vi "main-aq-program.vi"() -> ()   [LabVIEW 2015]
uses:
  <vilib>/userdefined/High Color/IMAQdx.ctl
  globals.vi
  <vilib>/vision/driver/NI_Vision_Acquisition_Software.lvlib
  <resource>/objmgr/imaqdx.rc
panel:
  in  "Save image":bool
  in  "Name":string
  in  "Path":path
  out "Image 2":T1(plugin-control)
  out "Image":T1(plugin-control)
  in  "Camera-right":T2="cam4"
  in  "Exposure time left":dbl=10000.0
  in  "Stop Button":bool
  in  "Camera-left":T2="cam4"
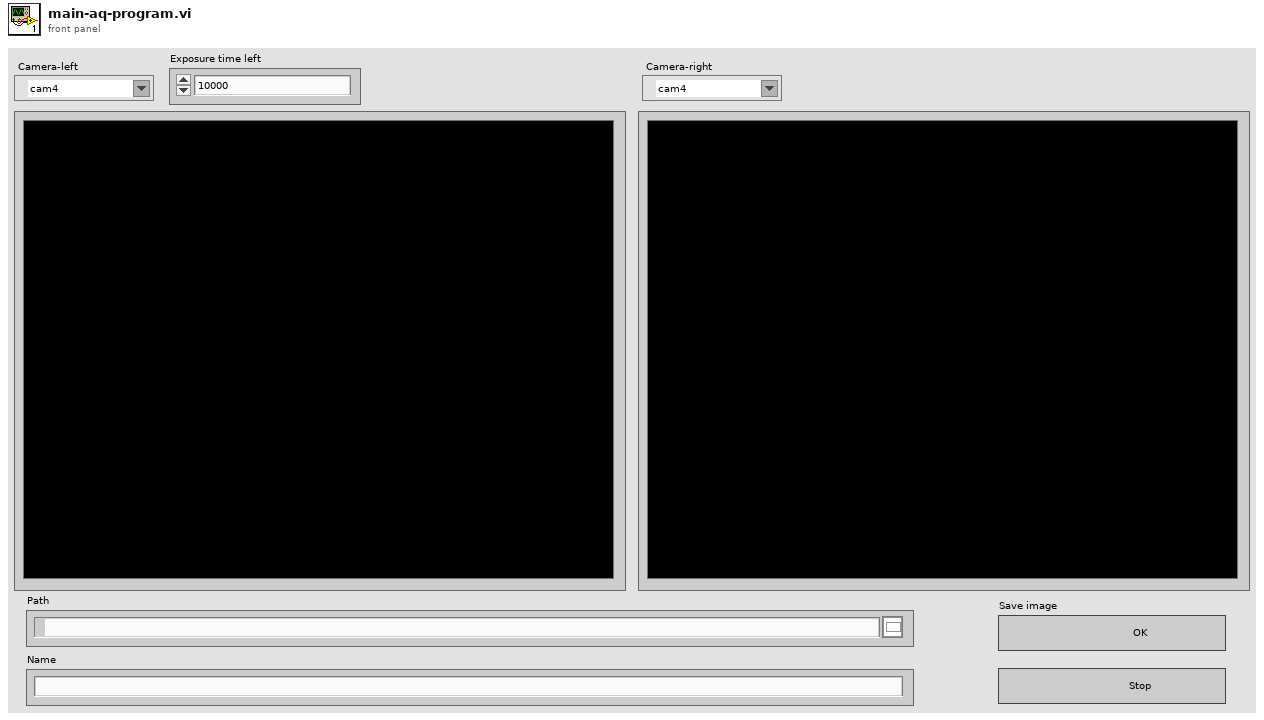
[diagram p1: front panel]
types:
  T1 = typedef "IMAQ Image.ctl" = refnum<image>
  T2 = typedef "IMAQdx.ctl" = refnum<k21>
  T3 = typedef "Image Type" = u32
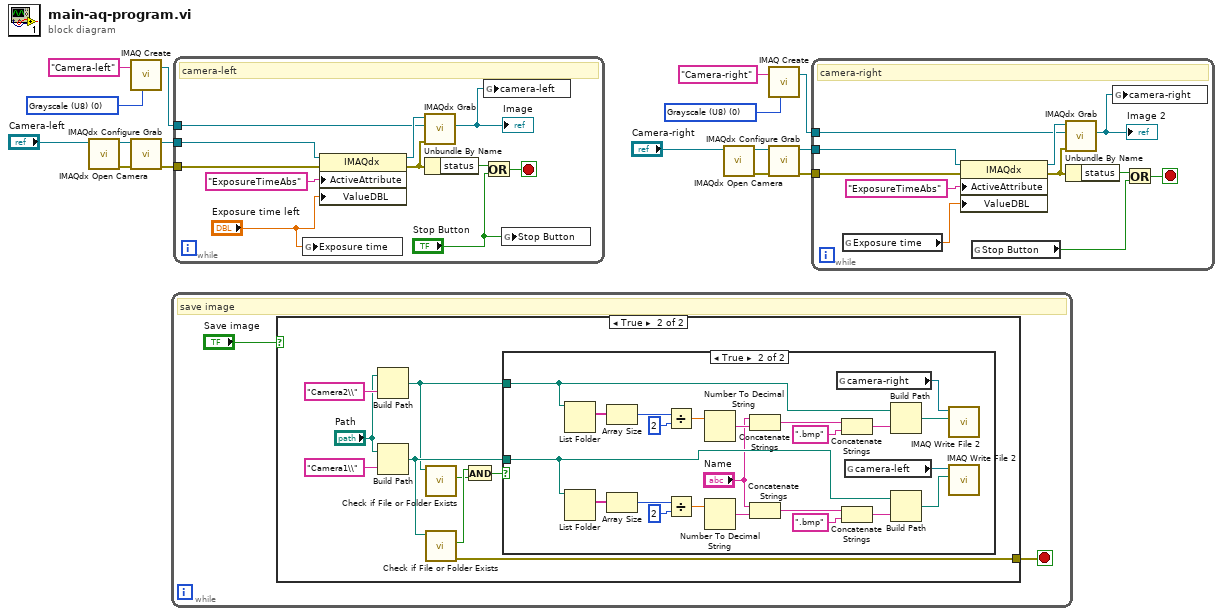
[diagram p0: block diagram]
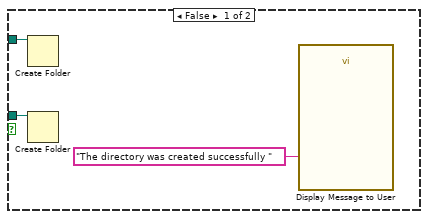
[diagram p3: hidden frame]
diagram:
  w10 = T3 0 items=["Grayscale (U8)", "Grayscale (I16)", "Grayscale (SGL)", "Complex (CSG)", "RGB (U32)", "HSL (U32)", "RGB (U64)"] ("Image Type")
  w16 = T3 0 items=["Grayscale (U8)", "Grayscale (I16)", "Grayscale (SGL)", "Complex (CSG)", "RGB (U32)", "HSL (U32)", "RGB (U64)"] ("Image Type")
  n1 = call <vilib>:"IMAQdx Open Camera.vi"("Session In"="Camera-left") -> ("error out"=w3:errorcluster, "Session Out"=w4:T2)  [unwired: 2 in, 7 out]
  n2 = call "IMAQ Create"("Image Name"="Camera-left", "Image Type"=w16) -> ("New Image"=w11:T1)  [unwired: 2 in, 2 out]
  n3 = call <vilib>:"IMAQdx Configure Grab.vi"("error in"=w3, "Session In"=w4) -> ("error out"=w12:errorcluster, "Session Out"=w13:T2)  [unwired: 8 out]
  n4 = while {
    stop <- w18 stop-if-true
    # "save image"
    n5 = case shown="True" "Save image" {
      tunnel: [_ w25] -> w18
      frame False {
      }
      frame True {
        n6 = Build Path(base path="Path", name or relative path="Camera2\\") -> (appended path=w20:path)
        n7 = Build Path(base path="Path", name or relative path="Camera1\\") -> (appended path=w26:path)
        n8 = call <vilib>:"Check if File or Folder Exists.vi"("path"=w20) -> ("file or folder exists?"=w22:bool)  [unwired: 8 in, 2 out]
        n9 = call <vilib>:"Check if File or Folder Exists.vi"("path"=w26) -> ("error out"=w25:errorcluster, "file or folder exists?"=w23:bool)  [unwired: 8 in, 1 out]
        n10 = And(x=w23, y=w22) -> (x .and. y?=w21:bool)
        n11 = case shown="True" w21 {
          tunnel: w26 -> [w30 w36]
          tunnel: w20 -> [w29 w37]
          frame False {
            n12 = Create Folder(path (use dialog)=w29) -> ()  [unwired: 2 in, 3 out]
            n13 = Create Folder(path (use dialog)=w30) -> ()  [unwired: 2 in, 3 out]
            n14 = call "Display Message to User"("Message"="The directory was created successfully ") -> ()  [unwired: 9 in, 2 out]
          }
          frame True {
            n15 = List Folder(path=w37) -> (filenames=w45:string[])  [unwired: 3 in, 3 out]
            n16 = List Folder(path=w36) -> (filenames=w53:string[])  [unwired: 3 in, 3 out]
            n17 = Array Size(array=w45) -> (size(s)=w44:i32)
            n18 = Array Size(array=w53) -> (size(s)=w52:i32)
            n19 = Divide(x=w44, y=2) -> (x/y=w42:dbl)
            n20 = Divide(x=w52, y=2) -> (x/y=w50:dbl)
            n21 = Number To Decimal String(number=w42) -> (decimal integer string=w41:string)  [unwired: 1 in]
            n22 = Number To Decimal String(number=w50) -> (decimal integer string=w49:string)  [unwired: 1 in]
            n23 = Concatenate Strings("Name", w41) -> (w40:string)
            n24 = Concatenate Strings("Name", w49) -> (w48:string)
            n25 = global read "globals.vi" "camera-right"() -> (w33:T1)
            n26 = Concatenate Strings(w40, ".bmp") -> (w38:string)
            n27 = Concatenate Strings(w48, ".bmp") -> (w46:string)
            n28 = global read "globals.vi" "camera-left"() -> (w31:T1)
            n29 = Build Path(base path=w37, name or relative path=w38) -> (appended path=w34:path)
            n30 = Build Path(base path=w36, name or relative path=w46) -> (appended path=w32:path)
            n31 = call-poly "IMAQ Write File 2"("File Path"=w34, "Image"=w33) -> ()  [unwired: 8 in, 2 out]
            n32 = call-poly "IMAQ Write File 2"("File Path"=w32, "Image"=w31) -> ()  [unwired: 8 in, 2 out]
          }
        }
      }
    }
  }
  n33 = while {
    tunnel: w13 -> [w59]
    tunnel: w12 -> [w58]
    tunnel: w11 -> [w57]
    stop <- w61 stop-if-true
    # "camera-left"
    n34 = global write "globals.vi" "Exposure time"("Exposure time left") -> ()
    n35 = property on="Property Node left" class="IMAQdx"(reference=w59, error in=w58, "ActiveAttribute"="ExposureTimeAbs" ("String"), "ValueDBL"="Exposure time left") -> (reference out=w63:T2, error out=w60:errorcluster)
    n36 = call <vilib>:"IMAQdx Grab.vi"("error in"=w60, "Image In"=w57, "Session In"=w63) -> ("Image Out"=w54:T1)  [unwired: 1 in, 7 out]
    "Image" <- w54
    n37 = Unbundle By Name(w60) -> ("status"=w62:bool)
    n38 = global write "globals.vi" "camera-left"(w54) -> ()
    n39 = Or(x=w62, y="Stop Button") -> (x .or. y?=w61:bool)
    n40 = global write "globals.vi" "Stop Button"("Stop Button") -> ()
  }
  n41 = call <vilib>:"IMAQdx Open Camera.vi"("Session In"="Camera-right") -> ("error out"=w1:errorcluster, "Session Out"=w2:T2)  [unwired: 2 in, 7 out]
  n42 = call "IMAQ Create"("Image Name"="Camera-right", "Image Type"=w10) -> ("New Image"=w5:T1)  [unwired: 2 in, 2 out]
  n43 = call <vilib>:"IMAQdx Configure Grab.vi"("error in"=w1, "Session In"=w2) -> ("error out"=w6:errorcluster, "Session Out"=w7:T2)  [unwired: 8 out]
  n44 = while {
    tunnel: w7 -> [w70]
    tunnel: w6 -> [w69]
    tunnel: w5 -> [w68]
    stop <- w72 stop-if-true
    # "camera-right"
    n45 = global read "globals.vi" "Exposure time"() -> (w66:dbl)
    n46 = property on="Property Node left" class="IMAQdx"(reference=w70, error in=w69, "ActiveAttribute"="ExposureTimeAbs" ("String"), "ValueDBL"=w66) -> (reference out=w74:T2, error out=w71:errorcluster)
    n47 = global read "globals.vi" "Stop Button"() -> (w67:bool)
    n48 = call <vilib>:"IMAQdx Grab.vi"("error in"=w71, "Image In"=w68, "Session In"=w74) -> ("Image Out"=w65:T1)  [unwired: 1 in, 7 out]
    "Image 2" <- w65
    n49 = Unbundle By Name(w71) -> ("status"=w73:bool)
    n50 = global write "globals.vi" "camera-right"(w65) -> ()
    n51 = Or(x=w73, y=w67) -> (x .or. y?=w72:bool)
  }
